vi "NFC - Read SN.vi"(7 "Python Version":string, 8 "error in (no error)":errorcluster, 11 "Reader SN":string="21121521200223") -> (0 "error out":errorcluster, 3 "Cartridge SN":string)   [LabVIEW 2020]
uses:
  Main/Main Globals.vi
panel:
  out "appended path":path
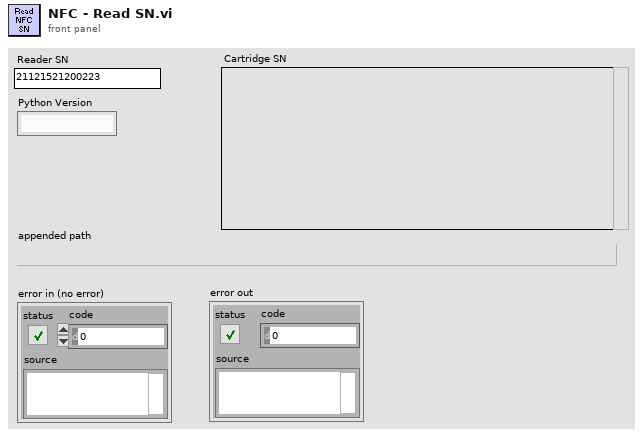
[diagram p1: front panel]
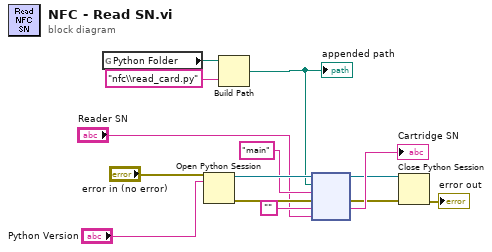
[diagram p0: block diagram]
diagram:
  n1 = global read "Main Globals.vi" "Python Folder"() -> (w4:path)
  n2 = Open Python Session(python version="Python Version", 3:"error in (no error)") -> (session out=w14:refnum<k35>, error out=w12:errorcluster)  [unwired: 1 in]
  n3 = Build Path(base path=w4, name or relative path="nfc\\read_card.py") -> (appended path=w2:path)
  "appended path" <- w2
  n4 = node(w14, w2, "main" ("function name"), w12, "" ("function name"), "Reader SN") -> (w8:refnum<k35>, w7:errorcluster, →"Cartridge SN":string)  [unwired: 1 in, 2 out]
  n5 = Close Python Session(session in=w8, error in=w7) -> (11:→"error out":errorcluster)
